vi "CSMKVMap-Write.vi"(8 "Error in":errorcluster caption="Error in (no error)", 10 "value":variant, 11 "name":string) -> (0 "Error out":errorcluster)   [LabVIEW 2017, in "Communicable State Machine.lvlib"]
uses:
  Communicable State Machine.lvlib
  _Support/ChangeFlag/ChangeFlag-Write.vi
  Utility/Random Change Flag.vi
  _Support/ChangeFlag/ChangeFlagDB.vi
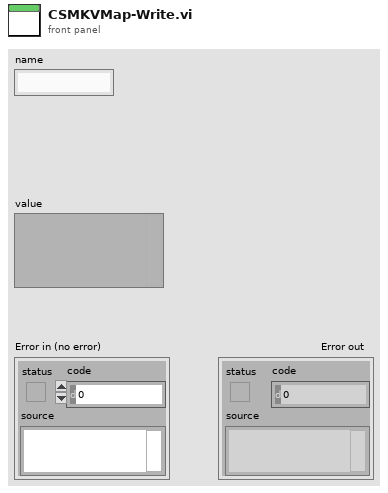
[diagram p1: front panel]
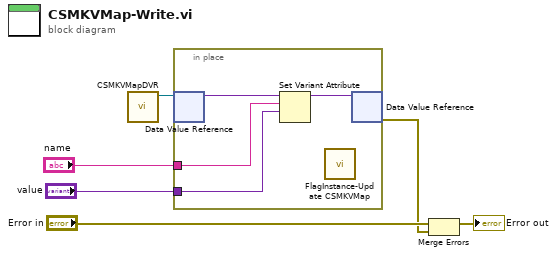
[diagram p0: block diagram]
diagram:
  n1 = call "CSMKVMapDVR.vi"() -> ("KVMapDVR"=w6:refnum<data-value>)  [unwired: 11 in]
  n2 = in-place {
    in-place-border: "name" -> [w8]
    in-place-border: "value" -> [w7]
    n3 = in-place-dvr #1(w6) -> (w10:variant)  [unwired: 1 out]
    n4 = Set Variant Attribute(Variant=w10, name=w8, value=w7) -> (Variant out=w9:variant)  [unwired: 1 in, 2 out]
    n5 = call "FlagInstance-Update CSMKVMap.vi"() -> ()  [unwired: 10 in, 2 out]
    n6 = in-place-dvr #1(w9) -> (w2:errorcluster)  [unwired: 1 out]
  }
  n7 = Merge Errors("Error in", w2) -> (→"Error out":errorcluster)
